vi "Test - New VI Object.vi"() -> ()   [LabVIEW 2019]
doc: "This VI is used by the New VI Object Location Argument.vi example."
panel:
  in  "Anchor 2":dbl
  in  "Anchor 1":dbl
  # "<------------ Point 100, 20"
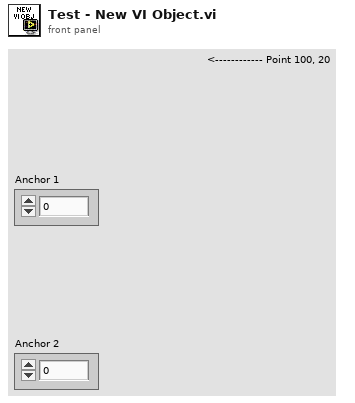
[diagram p1: front panel]
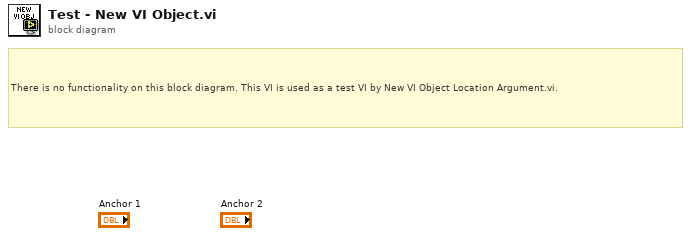
[diagram p0: block diagram]
diagram:
  # "There is no functionality on this block diagram. This VI is used as a test VI by New VI Object Location Argument.vi."
